vi "Register Job Event.vi"(11 "Job in":refnum<class "Job.lvclass">) -> (2 "Job Event Registration":refnum<event-registration>, 3 "Job out":refnum<class "Job.lvclass">)   [LabVIEW 2013, in "openCron.lvlib" / "Job.lvclass"]
uses:
  Job.lvclass
  Job Report -- cluster.ctl
  Job.lvclass/Job.ctl
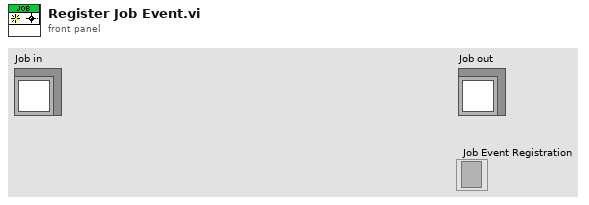
[diagram p1: front panel]
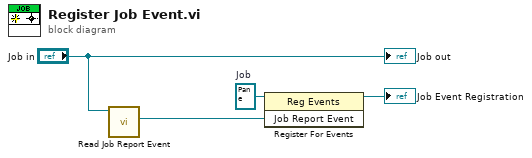
[diagram p0: block diagram]
diagram:
  w1 = refnum<event-registration> refnum  # Job
  n1 = call "Read Job Report Event.vi"("Job in"="Job in") -> ("Job Report Event"=w2:refnum<user-event>)  [unwired: 8 in, 2 out]
  n2 = register-events(reference=w1, w2) -> (reference out=→"Job Event Registration":refnum<event-registration>)  [unwired: 1 in, 1 out]
  "Job out" <- "Job in"
